vi "Set Pin.vi"(0 "NXP in":refnum<class "NXP.lvclass">, 5 "VISA resource name":refnum<visa-resource-name>, 7 "Pin":u8, 9 "Pin State":bool, 11 "error in (no error)":errorcluster) -> (4 "NXP out":refnum<class "NXP.lvclass">, 6 "VISA resource name 2":refnum<visa-resource-name>, 10 "String":string, 15 "error out":errorcluster)   [LabVIEW 2020, in "NXP.lvclass"]
uses:
  NXP.lvclass
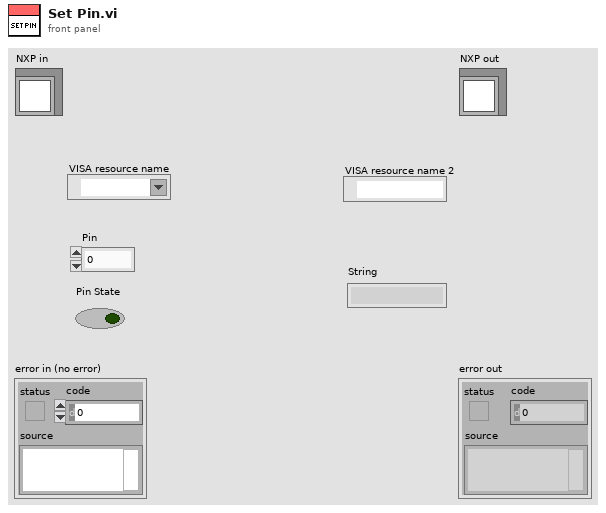
[diagram p1: front panel]
types:
  T1 = enum16{"Write", "Read", "Config", "Reset", "Close"}
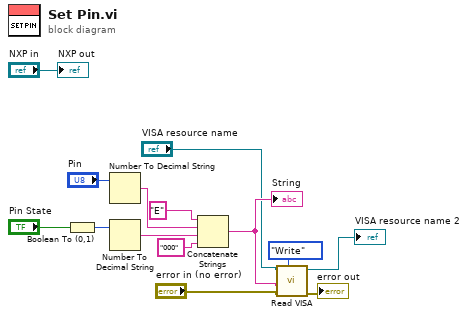
[diagram p0: block diagram]
diagram:
  n1 = Boolean To (0,1)(Boolean="Pin State") -> (0, 1=w9:i16)
  n2 = Number To Decimal String(number="Pin") -> (decimal integer string=w11:string)  [unwired: 1 in]
  n3 = Number To Decimal String(number=w9) -> (decimal integer string=w8:string)  [unwired: 1 in]
  n4 = Concatenate Strings("E" ("string"), w11, w8, "000" ("string")) -> (w4:string)
  "String" <- w4
  n5 = call "Read VISA.vi"("Opciones"=T1."Write", "error in (no error)"="error in (no error)", "Write"=w4, "VISA com port"="VISA resource name") -> ("error out"=→"error out":errorcluster, "VISA com port 2"=→"VISA resource name 2":refnum<visa-resource-name>)  [unwired: 5 in, 1 out]
  "NXP out" <- "NXP in"
